vi "Arm2Begin.vi"   [LabVIEW 2023]
doc: "Arm begin\nOpens ArmLift motor\nInputs:\nNone\nOutputs:\nnone"
uses:
  <vilib>/Rock Robotics/WPI/ThirdParty/REV Robotics/REVLib/Typedef/Spark MAX Sensor Type.ctl
  <vilib>/Rock Robotics/WPI/ThirdParty/REV Robotics/REVLib/Typedef/Spark MAX Limit Direction.ctl
  <vilib>/Rock Robotics/WPI/ThirdParty/REV Robotics/REVLib/Typedef/Spark MAX Limit Switch Polarity.ctl
  <vilib>/Rock Robotics/WPI/ThirdParty/REV Robotics/REVLib/Typedef/Spark MAX Idle Mode.ctl
  <vilib>/Rock Robotics/WPI/ThirdParty/REV Robotics/REVLib/Typedef/Spark MAX Motor Type.ctl
types:
  T1 = typedef "Spark MAX Sensor Type.ctl" = enum16{"No Sensor", "Hall Sensor", "Encoder", "-Not Available-", "Analog", "Alternate Encoder", "Duty Cycle"}
  T2 = typedef "Spark MAX Limit Switch Polarity.ctl" = enum16{"Normally Open", "Normally Closed"}
  T3 = typedef "Spark MAX Limit Direction.ctl" = enum16{"Forward Limit", "Reverse Limit"}
  T4 = typedef "Spark MAX Idle Mode.ctl" = enum16{"Coast", "Brake"}
  T5 = typedef "Spark MAX Motor Type.ctl" = enum16{"Brushed", "Brushless"}
  T6 = typedef "WPI_MotorControlDeviceRef.ctl" = cluster{"DeviceStatus":errorcluster, "Type":T7, "PWM":cluster{"PWM Channel":T8, "DeadBand":T9}, "CAN":cluster{"Device Number":u8, "SetOutput VI Ref":variant, "GetOutput VI Ref":variant, "Enable VI Ref":variant, "Disable VI Ref":variant, "Data":variant}, "Invert":bool, "DIO PWM":cluster{"PWM \"Enable\" Channel":T8, "DIOChannel":T10, "PWM Rate":dbl}}
  T7 = typedef "WPI_MotorControlType.ctl" = enum16{"PWM", "CAN", "DIO PWM"}
  T8 = typedef "FPGA_DIOPWMChannel.ctl" = enum8{"PWM 0", "PWM 1", "PWM 2", "PWM 3", "PWM 4", "PWM 5", "PWM 6", "PWM 7", "PWM 8", "PWM 9", "PWM MXP 0", "PWM MXP 1", "PWM MXP 2", "PWM MXP 3", "PWM MXP 4", "PWM MXP 5", "PWM MXP 6", "PWM MXP 7", "PWM MXP 8", "PWM MXP 9", "Invalid"}
  T9 = typedef "WPI_PWMDeadband.ctl" = cluster{"Name":string, "maxPositivePwm":i32, "minPositivePwm":i32, "centerPwm":i32, "maxNegativePwm":i32, "minNegativePwm":i32, "angularRange":u16}
  T10 = typedef "FPGA_DIOChannel.ctl" = enum8{"DIO 0", "DIO 1", "DIO 2", "DIO 3", "DIO 4", "DIO 5", "DIO 6", "DIO 7", "DIO 8", "DIO 9", "DIO MXP 0", "DIO MXP 1", "DIO MXP 2", "DIO MXP 3", "DIO MXP 4", "DIO MXP 5", "DIO MXP 6", "DIO MXP 7", "DIO MXP 8", "DIO MXP 9", "DIO MXP 10", "DIO MXP 11", "DIO MXP 12", "DIO MXP 13", "DIO MXP 14", "DIO MXP 15", "SPI Port CS1", "SPI Port CS2", "SPI Port CS3", "SPI Port MISO", "SPI Port MOSI", "Invalid"}
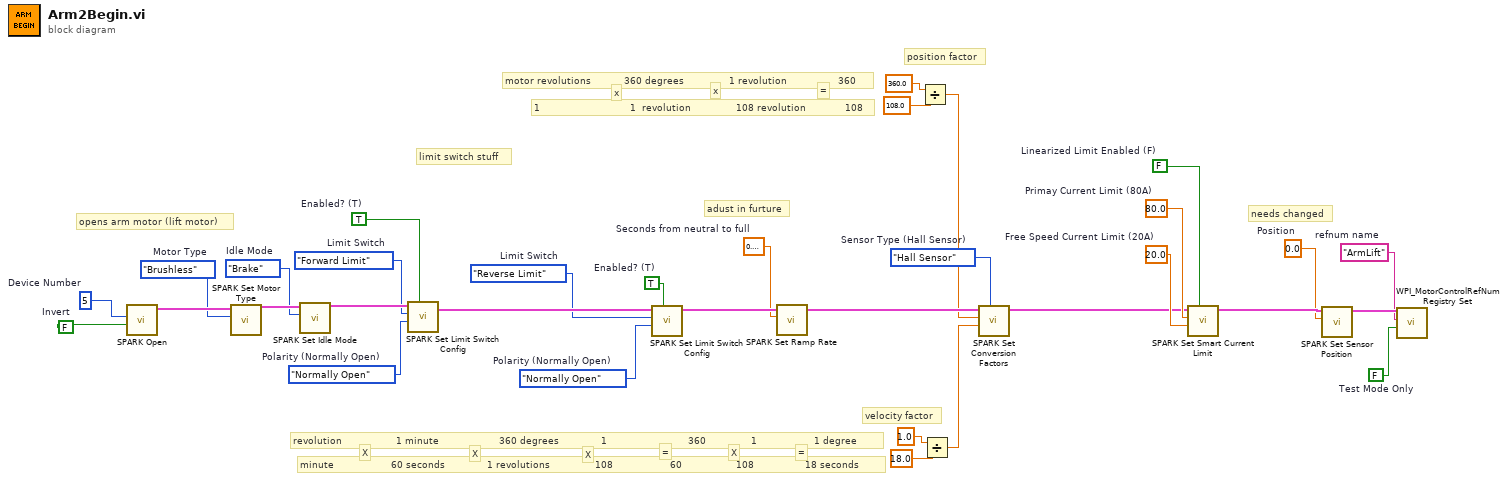
[diagram p0: block diagram]
diagram:
  w1 = FALSE  # Test Mode Only
  w8 = FALSE  # Linearized Limit Enabled (F)
  w10 = Spark_MAX_Sensor_Type."Hall Sensor"  # Sensor Type (Hall Sensor)
  w12 = sgl 0.2  # Seconds from neutral to full
  w14 = Spark_MAX_Limit_Switch_Polarity."Normally Open"  # Polarity (Normally Open)
  w15 = TRUE  # Enabled? (T)
  w16 = Spark_MAX_Limit_Direction."Reverse Limit"  # Limit Switch
  w18 = Spark_MAX_Limit_Switch_Polarity."Normally Open"  # Polarity (Normally Open)
  w19 = TRUE  # Enabled? (T)
  w20 = Spark_MAX_Limit_Direction."Forward Limit"  # Limit Switch
  w22 = 0.0  # Position
  w23 = "ArmLift"  # refnum name
  w26 = 20.0  # Free Speed Current Limit (20A)
  w27 = 80.0  # Primay Current Limit (80A)
  w28 = Spark_MAX_Idle_Mode."Brake"  # Idle Mode
  w30 = Spark_MAX_Motor_Type."Brushless"  # Motor Type
  w32 = FALSE  # Invert
  w33 = u8 5  # Device Number
  # "adust in furture"
  # "velocity factor"
  # "position factor"
  # "limit switch stuff"
  # "X"
  # "X"
  # "X"
  # "X"
  # "="
  # "="
  # "minute                   60 seconds              1 revolutions               108                   60                  108                 18 seconds"
  # "revolution                  1 minute                    360 degrees              1                           360               1                   1 degree"
  # "1                              1  revolution               108 revolution             108"
  # "="
  # "x"
  # "x"
  # "motor revolutions           360 degrees               1 revolution                 360"
  # "needs changed"
  # "opens arm motor (lift motor)"
  n1 = call <vilib>:"SPARK Open.vi"("Invert"=w32, "Device Number"=w33) -> ("MotorControlDeviceRef"=w31:T6)  [unwired: 8 in, 1 out]
  n2 = call <vilib>:"SPARK Set Motor Type.vi"("Motor Type"=w30, "MotorControlDevRef"=w31) -> ("MotorControlDeviceRef"=w29:T6)  [unwired: 8 in, 1 out]
  n3 = call <vilib>:"SPARK Set Idle Mode.vi"("Idle Mode"=w28, "MotorControlDeviceRef in"=w29) -> ("MotorControlDeviceRef out"=w21:T6)  [unwired: 8 in, 1 out]
  n4 = call <vilib>:"SPARK Set Limit Switch Config.vi"("Enabled? (T)"=w19, "Polarity (Normally Open)"=w18, "Limit Switch"=w20, "MotorControlDeviceRef in"=w21) -> ("MotorControlDeviceRef out"=w17:T6)  [unwired: 6 in, 1 out]
  n5 = call <vilib>:"SPARK Set Limit Switch Config.vi"("Enabled? (T)"=w15, "Polarity (Normally Open)"=w14, "Limit Switch"=w16, "MotorControlDeviceRef in"=w17) -> ("MotorControlDeviceRef out"=w13:T6)  [unwired: 6 in, 1 out]
  n6 = call <vilib>:"SPARK Set Ramp Rate.vi"("Seconds from neutral to full (0)"=w12, "MotorControlDeviceRef in"=w13) -> ("MotorControlDeviceRef"=w11:T6)  [unwired: 8 in, 1 out]
  n7 = Divide(x=360.0 ("Velocity Factor (1)"), y=108.0) -> (x/y=w2:dbl)
  n8 = Divide(x=1.0 ("Velocity Factor (1)"), y=18.0) -> (x/y=w7:dbl)
  n9 = call <vilib>:"SPARK Set Conversion Factors.vi"("Sensor Type (Hall Sensor)"=w10, "Velocity Factor (1)"=w7, "Position Factor (1)"=w2, "MotorControlDeviceRef in"=w11) -> ("MotorControlDeviceRef out"=w9:T6)  [unwired: 6 in, 1 out]
  n10 = call <vilib>:"SPARK Set Smart Current Limit.vi"("Linearized Limit Enabled (F)"=w8, "Free Speed Current Limit (20A)"=w26, "Primay Current Limit (80A)"=w27, "MotorControlDeviceRef in"=w9) -> ("MotorControlDeviceRef out"=w25:T6)  [unwired: 6 in, 1 out]
  n11 = call <vilib>:"SPARK Set Sensor Position.vi"("Position"=w22, "MotorControlDeviceRef"=w25) -> ("MotorControlDeviceRef"=w24:T6)  [unwired: 8 in, 1 out]
  n12 = call <vilib>:"WPI_MotorControlRefNum Registry Set.vi"("Test Mode Only"=w1, "refnum name"=w23, "MotorControlDevRef"=w24) -> ()  [unwired: 7 in, 2 out]
